vi "On Click Cancel Camera Calibration.vi"(8 "error in (no error)":errorcluster, 11 "App in":refnum<class "App.lvclass">) -> (0 "error out":errorcluster, 3 "App out":refnum<class "App.lvclass">)   [LabVIEW 2020, in "AR Example.lvlib" / "App.lvclass"]
uses:
  App.lvclass
  App.lvclass/App.ctl
  UI/UI.lvclass
  UI/Tab Control.ctl
  Timeout Action.ctl
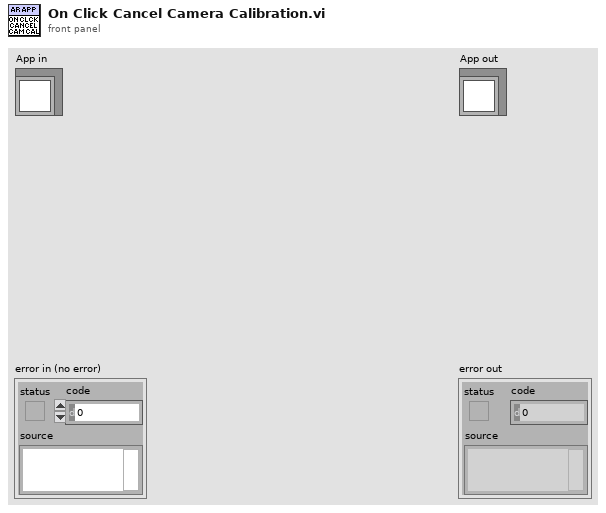
[diagram p1: front panel]
types:
  T1 = typedef "AR Example.lvlib/App.lvclass/Timeout Action.ctl" = enum16{"None", "Setup Camera Action", "Camera Calibration Action"}
  T2 = typedef "AR Example.lvlib/UI.lvclass/Tab Control.ctl" = enum8{"Config Load", "Camera Selection", "Camera Calibration"}
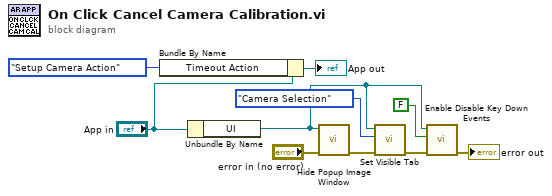
[diagram p0: block diagram]
diagram:
  n1 = Bundle By Name(cluster="App in", "Timeout Action"=Timeout_Action."Setup Camera Action" ("Shared.Timeout Action")) -> (→"App out":refnum<class "App.lvclass">)
  n2 = Unbundle By Name("App in") -> ("UI"=w2:refnum<class "UI.lvclass">)
  n3 = call "Hide Popup Image Window.vi"("error in (no error)"="error in (no error)", "UI in"=w2) -> ("error out"=w8:errorcluster)  [unwired: 9 in]
  n4 = call-dynamic "Set Visible Tab.vi"("error in (no error)"=w8, "Value"=Tab_Control."Camera Selection", "UI in"=w2) -> ("error out"=w7:errorcluster)  [unwired: 8 in]
  n5 = call "Enable Disable Key Down Events.vi"("error in (no error)"=w7, "Enable?"=FALSE, "UI in"=w2) -> ("error out"=→"error out":errorcluster)  [unwired: 8 in]
